vi "GraphView.vi"() -> ()   [LabVIEW 2014]
uses:
  <vilib>/Utility/miscctls.llb/LVCursorListTypeDef.ctl
  GlobalData/GlobalData.vi
panel:
  out "波形グラフ":waveform(dbl)[](graph)
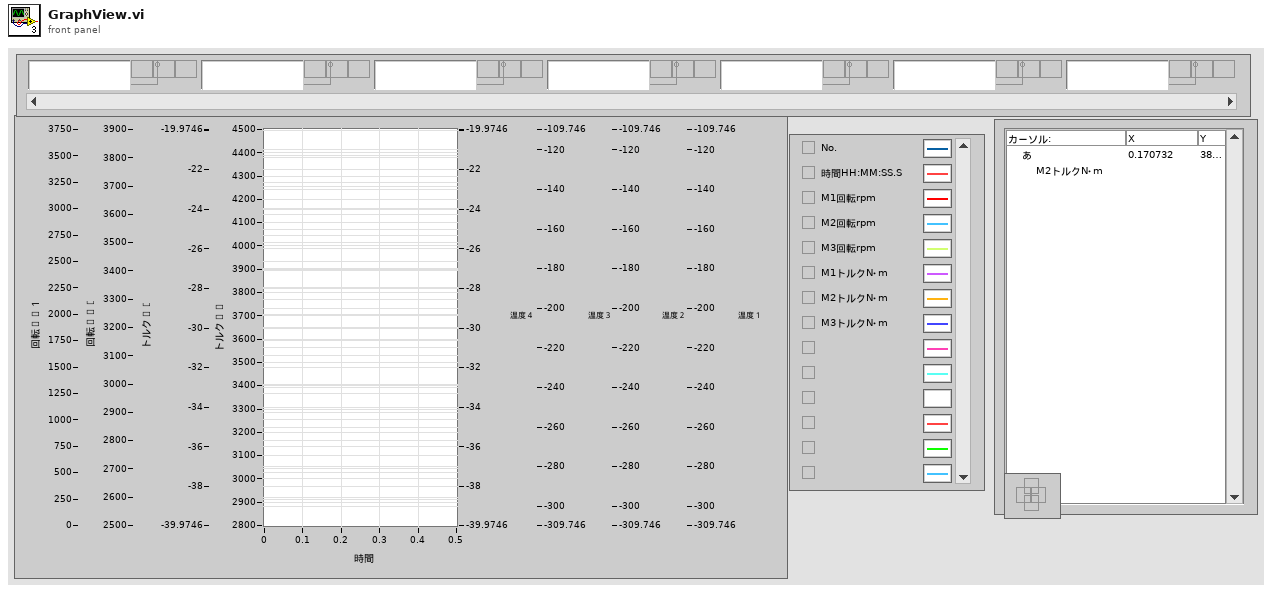
[diagram p1: front panel]
types:
  T1 = typedef "LVCursorListTypeDef.ctl" = cluster{"Name":string, "Color":u32, "Style":u8, "Point Style":u8, "Name Visible":bool, "Allow Drag":bool, "Cursor Mode":u32, "Plot":i32, "Index":i32, "Position":cluster{"X":dbl, "Y":dbl}, "X Scale":u32, "Y Scale":u32, "Watch Plots":i32[], "Watch All Plots":bool, "Plot Area":i32, "Label Offset":cluster{"X":dbl, "Y":dbl}}[]
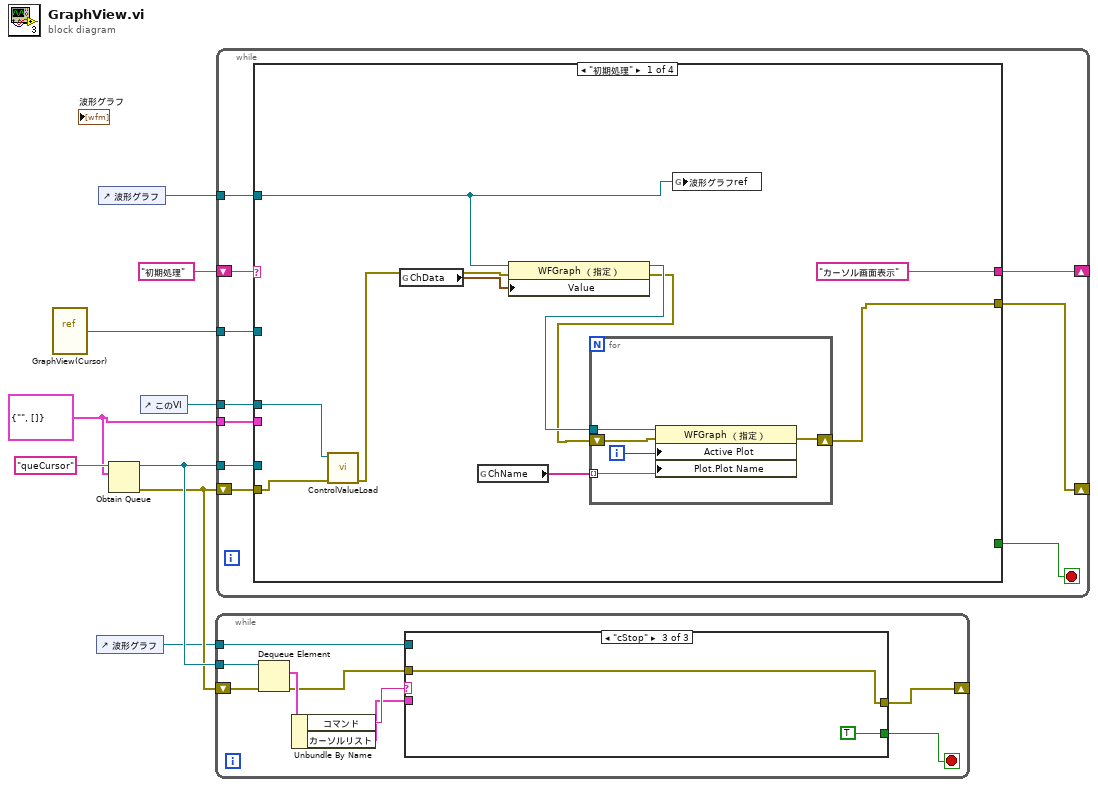
[diagram p0: block diagram]
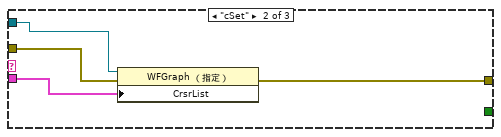
[diagram p3: hidden frame]
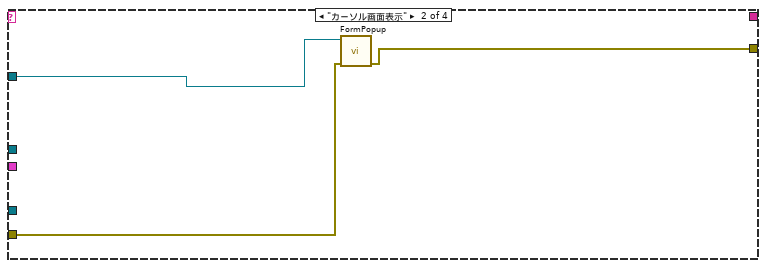
[diagram p4: hidden frame]
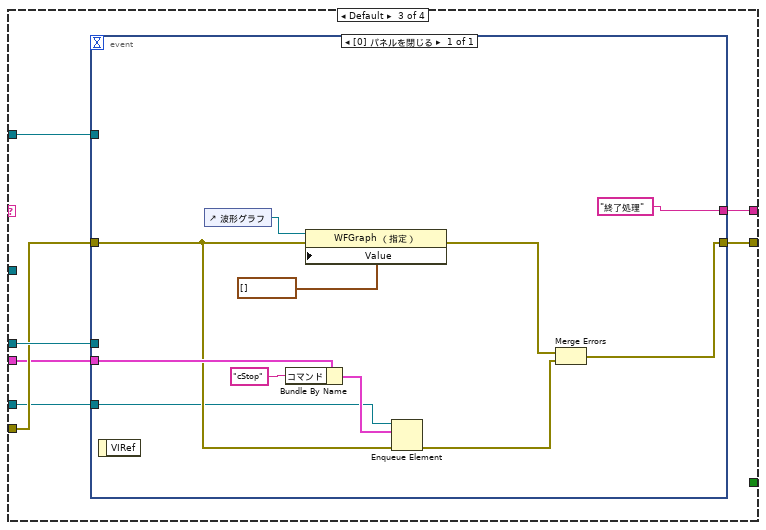
[diagram p5: hidden frame]
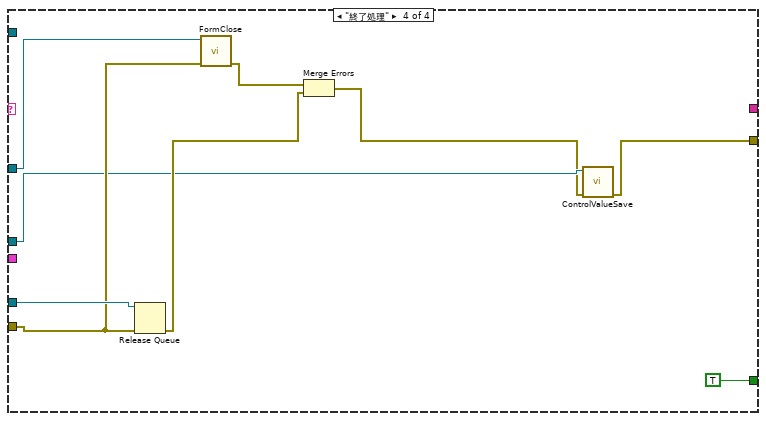
[diagram p6: hidden frame]
diagram:
  w5 = cluster{"コマンド":string, "カーソルリスト":T1} {"コマンド"="", "カーソルリスト"=[]}
  n1 = vi-ref "GraphView(Cursor).vi"() -> (w1:refnum<vi>)
  n2 = control-ref of="波形グラフ"() -> (w2:refnum<vi>)
  n3 = control-ref of="波形グラフ"() -> (w8:refnum<vi>)
  n4 = Obtain Queue(name (unnamed)="queCursor" ("名前（名前なし）"), element data type=w5) -> (queue out=w4:refnum<queue>, error out=w3:errorcluster)  [unwired: 3 in, 1 out]
  n5 = control-ref of="このVI"() -> (w9:refnum<vi>)
  n6 = while {
    tunnel: w4 -> [w18]
    shift-right: [w11] -> _
    shift-left: w3 -> [w17]
    tunnel: w2 -> [w13]
    stop <- w10 stop-if-true
    n7 = Dequeue Element(queue=w18, error in (no error)=w17) -> (element=w16:cluster{"コマンド":string, "カーソルリスト":T1}, error out=w12:errorcluster)  [unwired: 1 in, 2 out]
    n8 = Unbundle By Name(w16) -> ("コマンド"=w15:string, "カーソルリスト"=w14:T1)
    n9 = case shown="\"cStop\"" w15 {
      tunnel: w14 -> [_ w20 _]
      tunnel: w13 -> [_ w23 _]
      tunnel: w12 -> [w19 w22 w24]
      tunnel: [w19 w21 w24] -> w11
      tunnel: [_ _ TRUE] -> w10
      frame Default {
      }
      frame "cSet" {
        n10 = property class="WFGraph （指定）"(reference=w23, error in=w22, "CrsrList"=w20) -> (error out=w21:errorcluster)  [unwired: 1 out]
      }
      frame "cStop" {
      }
    }
  }
  n11 = while {
    tunnel: w9 -> [w35]
    shift-right: [w33] -> _
    shift-left: w3 -> [w34]
    tunnel: w8 -> [w32]
    shift-right: [w29] -> _
    shift-left: "初期処理" -> [w30]
    tunnel: w4 -> [w31]
    tunnel: w5 -> [w28]
    tunnel: w1 -> [w26]
    stop <- w27 stop-if-true
    n12 = case shown="\"初期処理\"" w30 {
      tunnel: w35 -> [w42 _ w60 w74]
      tunnel: w34 -> [w45 w53 w59 w77]
      tunnel: [w36 w52 w58 w72] -> w33
      tunnel: w32 -> [w41 _ w57 _]
      tunnel: w31 -> [_ _ w56 w80]
      tunnel: ["カーソル画面表示" _ w55 _] -> w29
      tunnel: w28 -> [_ _ w54 _]
      tunnel: [_ _ _ TRUE] -> w27
      tunnel: w26 -> [_ w51 _ w78]
      frame "初期処理" {
        n13 = call "ControlValueLoad.vi"("err(in)"=w45, "VI refnum"=w42) -> ("err(out)"=w43:errorcluster)  [unwired: 9 in]
        n14 = global read "GlobalData.vi" "ChData"() -> (w44:waveform(dbl)[])
        n15 = global read "GlobalData.vi" "ChName"() -> (w39:string[])
        n16 = property class="WFGraph （指定）"(reference=w41, error in=w43, "Value"=w44) -> (reference out=w38:refnum<vi>, error out=w37:errorcluster)
        n17 = for {
          tunnel: w38 -> [w50]
          tunnel: w39 -> [w49] mode=indexing
          shift-right: [w46] -> w36
          shift-left: w37 -> [w47]
          i -> [w48]
          n18 = property class="WFGraph （指定）"(reference=w50, error in=w47, "Active Plot"=w48, "Plot.Plot Name"=w49) -> (error out=w46:errorcluster)  [unwired: 1 out]
        }
        n19 = global write "GlobalData.vi" "波形グラフref"(w41) -> ()
      }
      frame "カーソル画面表示" {
        n20 = call "FormPopup.vi"("エラー入力（エラーなし）"=w53, "VI入力"=w51) -> ("エラー出力"=w52:errorcluster)  [unwired: 9 in]
      }
      frame Default {
        n21 = event shown="[0] パネルを閉じる" {
          selector: _ -> [_]
          dyn-events: _ -> [_]
          timeout: _ -> [_]
          tunnel: w60 -> [_]
          tunnel: w59 -> [w65]
          tunnel: [w63] -> w58
          tunnel: w57 -> [_]
          tunnel: w56 -> [w61]
          tunnel: ["終了処理"] -> w55
          tunnel: w54 -> [w68]
          event Panel Close {
            n22 = event-data() -> ()  [unwired: 1 in, 1 out]
            n23 = control-ref of="波形グラフ"() -> (w71:refnum<vi>)
            n24 = Bundle By Name(cluster=w68, "コマンド"="cStop") -> (w66:cluster{"コマンド":string, "カーソルリスト":T1})
            n25 = property class="WFGraph （指定）"(reference=w71, error in=w65, "Value"=waveform(dbl)[] [] ("値")) -> (error out=w64:errorcluster)  [unwired: 1 out]
            n26 = Enqueue Element(queue=w61, element=w66, error in (no error)=w65) -> (error out=w62:errorcluster)  [unwired: 1 in, 2 out]
            n27 = Merge Errors(w64, w62) -> (w63:errorcluster)
          }
        }
      }
      frame "終了処理" {
        n28 = Release Queue(queue=w80, error in (no error)=w77) -> (error out=w75:errorcluster)  [unwired: 1 in, 2 out]
        n29 = call "FormClose.vi"("エラー入力（エラーなし）"=w77, "VI入力"=w78) -> ("エラー出力"=w76:errorcluster)  [unwired: 9 in]
        n30 = Merge Errors(w76, w75) -> (w73:errorcluster)
        n31 = call "ControlValueSave.vi"("err(in)"=w73, "VI refnum"=w74) -> ("err(out)"=w72:errorcluster)  [unwired: 9 in]
      }
    }
  }
